vi "MessageBox.vi"(8 "Error In":errorcluster, 11 "Message":string) -> (0 "Error Out":errorcluster)   [LabVIEW 2018]
panel:
  out "String Indicator":string
  in  "OK Button":bool
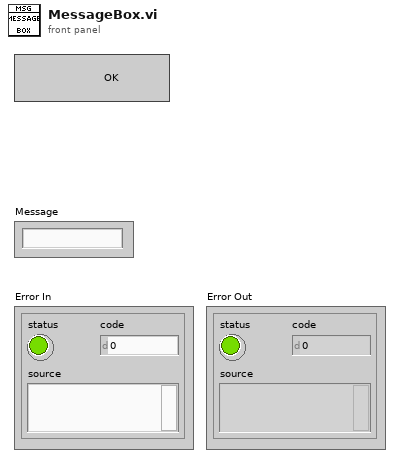
[diagram p1: front panel]
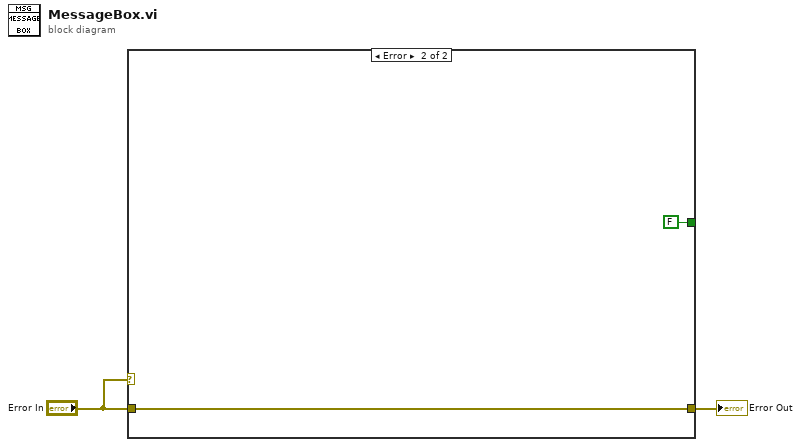
[diagram p0: block diagram]
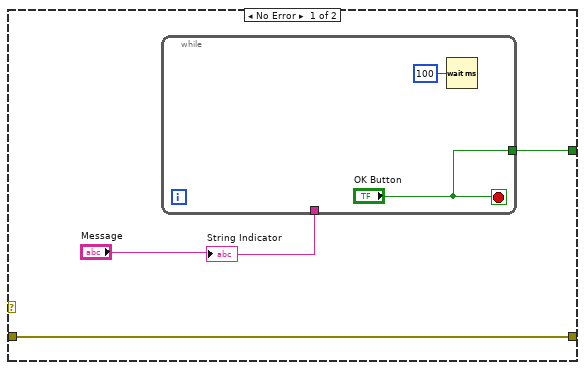
[diagram p2: hidden frame]
diagram:
  n1 = case shown="Error" "Error In" {
    tunnel: "Error In" -> [w4 w8]
    tunnel: [w4 w8] -> w1
    tunnel: [w3 FALSE ("OK Button")] -> _
    frame No Error {
      n2 = while {
        tunnel: "Message" -> [_]
        tunnel: ["OK Button"] -> w3
        stop <- "OK Button" stop-if-true
        n3 = Wait (ms)(milliseconds to wait=u32 100) -> ()  [unwired: 1 out]
      }
      "String Indicator" <- "Message"
    }
    frame Error {
    }
  }
  "Error Out" <- w1
